vi "Init DAQ.vi"(8 "error in":errorcluster, 11 "Notifiers in":T1) -> (0 "error out":errorcluster, 3 "Notifiers out":T1)   [LabVIEW 2015, in "DAQ.lvlib"]
uses:
  DAQ.lvlib
  support/Notifiers/Notifiers.ctl
  support/Message Queue/Enqueue Message (Single).vi
  support/Message Queue/Message Queue.lvlib
  PLC/PLC.lvlib
  Support/Notifiers/Notifiers.lvlib
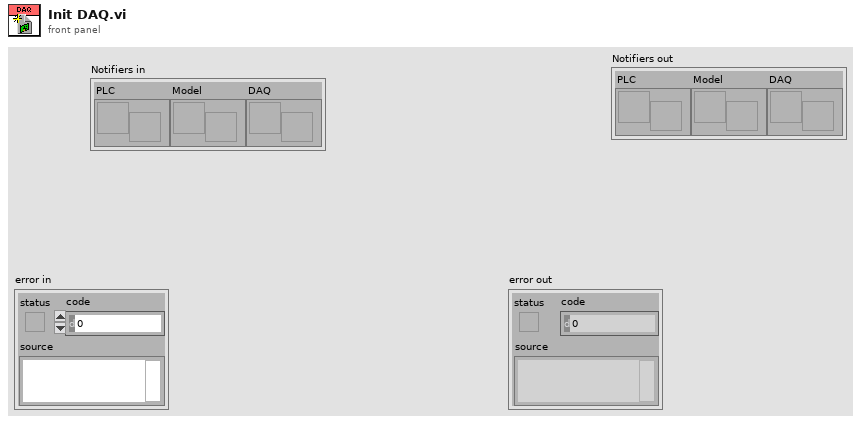
[diagram p1: front panel]
types:
  T1 = typedef "Notifiers.lvlib/Notifiers.ctl" = cluster{"PLC":refnum<notifier>, "Model":refnum<notifier>, "DAQ":refnum<notifier>}
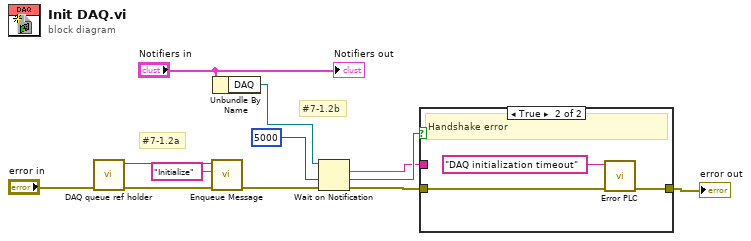
[diagram p0: block diagram]
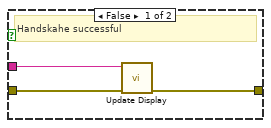
[diagram p2: hidden frame]
diagram:
  # "#7-1.2b"
  # "#7-1.2a"
  n1 = call "DAQ queue ref holder.vi"("error in"="error in") -> ("error out"=w5:errorcluster, "Input Message Queue"=w4:refnum<queue>)  [unwired: 9 in]
  n2 = call-poly "Enqueue Message.vi"("error in (no error)"=w5, "Message"="Initialize", "Message Queue"=w4) -> ("error out"=w8:errorcluster)  [unwired: 7 in, 1 out]
  n3 = Unbundle By Name("Notifiers in") -> ("DAQ"=w1:refnum<notifier>)
  n4 = Wait on Notification(notifier=w1, timeout in ms (-1)=5000, error in (no error)=w8) -> (notification=w7:string, timed out?=w10:bool, error out=w11:errorcluster)  [unwired: 1 in, 1 out]
  n5 = case shown="True" w10 {
    tunnel: w11 -> [w14 w17]
    tunnel: [w13 w16] -> w12
    tunnel: w7 -> [w15 _]
    frame False {
      # "Handskahe successful"
      n6 = call "Update Display.vi"("error in"=w14, "Message string"=w15) -> ("error out"=w13:errorcluster)  [unwired: 9 in]
    }
    frame True {
      # "Handshake error"
      n7 = call "Error PLC.vi"("error in"=w17, "String"="DAQ initialization timeout" ("Message")) -> ("error out"=w16:errorcluster)  [unwired: 9 in]
    }
  }
  "error out" <- w12
  "Notifiers out" <- "Notifiers in"
